vi "PWM Write.vi"(8 "error in":errorcluster, 9 "Duty Cycle":dbl, 10 "Frequency":dbl, 11 "FPGA Interface":refnum<k20>) -> (0 "error out":errorcluster)   [LabVIEW 2013, in "PWM Engine.lvlib"]
uses:
  PWM Engine.lvlib
  <vilib>/rvi/interface/common/niFpgaWaitOnOcc.vi
  <vilib>/Utility/error.llb/Error Cluster From Error Code.vi
  <vilib>/rvi/errors/niLvFpgaAdjustHostInterfaceError.vi
  <vilib>/rvi/interface/nirviReadWriteControl/nirviReadWriteControl.xnode
  NiFpgaLv.dll
  <vilib>/rvi/interface/Simulation/niFpgaSimulationCallBeginRW.vi
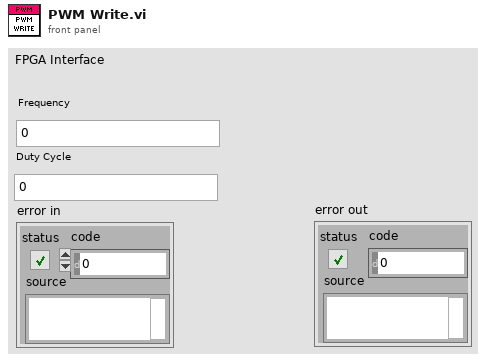
[diagram p1: front panel]
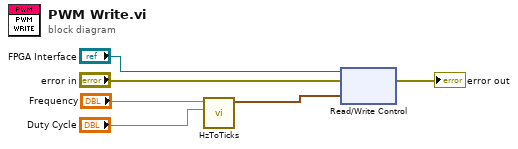
[diagram p0: block diagram]
diagram:
  n1 = call "HzToTicks.vi"("Duty Cycle"="Duty Cycle", "Frequency"="Frequency") -> ("Ticks"=w6:cluster{"Low Ticks":u32, "High Ticks":u32})  [unwired: 9 in]
  n2 = xnode "Read/Write Control"("FPGA VI Reference In"="FPGA Interface", "error in"="error in", "Value"=w6) -> ("error out"=→"error out":errorcluster)  [unwired: 1 out]
